vi "RetVal.vi"() -> ()   [LabVIEW 2017]
panel:
  out "RetVal":bool
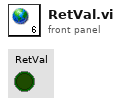
[diagram p1: front panel]
diagram:
